vi "保存流水号.vi"(8 "error in":errorcluster, 10 "流水号":dbl) -> (0 "error out":errorcluster)   [LabVIEW 2016]
uses:
  <vilib>/Utility/config.llb/Write Key (Double).vi
  <vilib>/Utility/config.llb/NI_LVConfig.lvlib
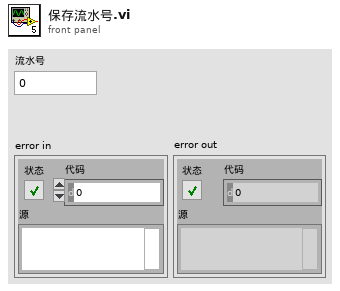
[diagram p1: front panel]
types:
  T1 = cluster{"CalData":path, "Datasave":path, "Data":path}
  T2 = typedef "NI_LVConfig.lvlib/Config Data RefNum.ctl" = refnum<k1>
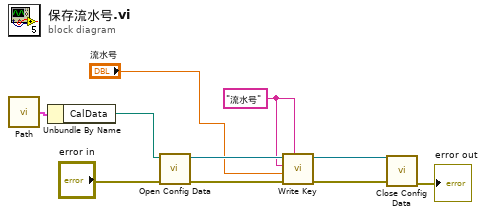
[diagram p0: block diagram]
diagram:
  w6 = "流水号"
  n1 = call "Path.vi"() -> ("path"=w5:T1)  [unwired: 9 in]
  n2 = Unbundle By Name(w5) -> ("CalData"=w4:path)
  n3 = call <vilib>:"Open Config Data.vi"("error in (no error)"="error in", "configuration file path"=w4) -> ("error out"=w10:errorcluster, "refnum"=w7:T2)  [unwired: 7 in, 1 out]
  n4 = call-poly <vilib>:"Write Key.vi"("section"=w6, "error in (no error)"=w10, "value"="流水号", "key"=w6, "refnum"=w7) -> ("error out"=w9:errorcluster, "refnum out"=w8:T2)  [unwired: 4 in, 1 out]
  n5 = call <vilib>:"Close Config Data.vi"("error in (no error)"=w9, "refnum"=w8) -> ("error out"=→"error out":errorcluster)  [unwired: 8 in, 1 out]
